vi "LoopselFF_1_or_2cam_eventdriven_CC.VI"() -> ()   [LabVIEW 2015]
uses:
  board.vis/Globals.vi
  <vilib>/Analysis/NI_AALBase.lvlib
panel:
  in  "channel select\n1: CHA\n2: CHB\n3: both CH":u16=3
  out "tRMS":dbl=8.272957184592048 format="%0#.1f"
  out "mean":dbl=3064.5285285285286 format="%#_4f"
  in  "Pixel":u16=100
  in  "is FFT":bool=TRUE
  in  "IR gain":bool
  in  "continuous":bool=TRUE
  out "curr.block":u8=1
  out "Measure ON":bool
  in  "Board select\n1: board 1\n2: board 2\n3: both boards":u8=3
  in  "no.of blocks (nob)\npress enter":u32=1
  in  "NOB":u32(slide)=1 max=10 scale=0.9..1.0
  out "Signalverlaufgraph 2":u16[](graph)=[0, 0, 543, 543, 0, 1, 0, 0, 2, 2, 3, 3, 4, 4, 5, 5, 6, 6, 7, 7, 8, 8, 9, 9, 10, 10, 11, 11, 12, 12, 13, 13, 14, 14, 15, 15, 16, 16, 17, 17, 18, 18, 19, 19, 20, 20, 21, 21, 22, 22, 23, 23, 24, 24, 25, 25, 26, 26, 27, 27, 28, 28, 29, 29, 30, 30, 31, 31, 32, 32, 33, 33, 34, 34, 35, 35, 36, 36, 37, 37, 38, 38, 39, 39, 40, 40, 41, 41, 42, 42, 43, 43, 44, 44, 45, 45, 46, 46, 47, 47, 48, 48, 49, 49, 50, 50, 51, 51, 52, 52, 53, 53, 54, 54, 55, 55, 56, 56, 57, 57, 58, 58, 59, 59, 60, 60, 61, 61, 62, 62, 63, 63, 64, 64, 65, 65, 66, 66, 67, 67, 68, 68, 69, 69, 70, 70, 71, 71, 72, 72, 73, 73, 74, 74, 75, 75, 76, 76, 77, 77, 78, 78, 79, 79, 80, 80, 81, 81, 82, 82, 83, 83, 84, 84, 85, 85, 86, 86, 87, 87, 88, 88, 89, 89, 90, 90, 91, 91, 92, 92, 93, 93, 94, 94, 95, 95, 96, 96, 97, 97, 98, 98, 99, 99, 100, 100, 101, 101, 102, 102, 103, 103, 104, 104, 105, 105, 106, 106, 107, 107, 108, 108, 109, 109, 110, 110, 111, 111, 112, 112, 113, 113, 114, 114, 115, 115, 116, 116, 117, 117, 118, 118, 119, 119, 120, 120, 121, 121, 122, 122, 123, 123, 124, 124, 125, 125, 126, 126, 127, 127, 128, 128, 129, 129, 130, 130, 131, 131, 132, 132, 133, 133, 134, 134, 135, 135, 136, 136, 137, 137, 138, 138, 139, 139, 140, 140, 141, 141, 142, 142, 143, 143, 144, 144, 145, 145, 146, 146, 147, 147, 148, 148, 149, 149, 150, 150, 151, 151, 152, 152, 153, 153, 154, 154, 155, 155, 156, 156, 157, 157, 158, 158, 159, 159, 160, 160, 161, 161, 162, 162, 163, 163, 164, 164, 165, 165, 166, 166, 167, 167, 168, 168, 169, 169, 170, 170, 171, 171, 172, 172, 173, 173, 174, 174, 175, 175, 176, 176, 177, 177, 178, 178, 179, 179, 180, 180, 181, 181, 182, 182, 183, 183, 184, 184, 185, 185, 186, 186, 187, 187, 188, 188, 189, 189, 190, 190, 191, 191, 192, 192, 193, 193, 194, 194, 195, 195, 196, 196, 197, 197, 198, 198, 199, 199, 200, 200, 201, 201, 202, 202, 203, 203, 204, 204, 205, 205, 206, 206, 207, 207, 208, 208, 209, 209, 210, 210, 211, 211, 212, 212, 213, 213, 214, 214, 215, 215, 216, 216, 217, 217, 218, 218, 219, 219, 220, 220, 221, 221, 222, 222, 223, 223, 224, 224, 225, 225, 226, 226, 227, 227, 228, 228, 229, 229, 230, 230, 231, 231, 232, 232, 233, 233, 234, 234, 235, 235, 236, 236, 237, 237, 238, 238, 239, 239, 240, 240, 241, 241, 242, 242, 243, 243, 244, 244, 245, 245, 246, 246, 247, 247, 248, 248, 249, 249, 250, 250, 251, 251, 252, 252, 253, 253, 254, 254, 255, 255, 256, 256, 257, 257, 258, 258, 259, 259, 260, 260, 261, 261, 262, 262, 263, 263, 264, 264, 265, 265, 266, 266, 267, 267, 268, 268, 269, 269, 270, 270, 271, 271, 272, 272, 273, 273, 274, 274, 275, 275, 276, 276, 277, 277, 278, 278, 279, 279, 280, 280, 281, 281, 282, 282, 283, 283, 284, 284, 285, 285, 286, 286, 287, 287, 288, 288, 289, 289, 290, 290, 291, 291, 292, 292, 293, 293, 294, 294, 295, 295, 296, 296, 297, 297, 298, 298, 299, 299, 300, 300, 301, 301, 302, 302, 303, 303, 304, 304, 305, 305, 306, 306, 307, 307, 308, 308, 309, 309, 310, 310, 311, 311, 312, 312, 313, 313, 314, 314, 315, 315, 316, 316, 317, 317, 318, 318, 319, 319, 320, 320, 321, 321, 322, 322, 323, 323, 324, 324, 325, 325, 326, 326, 327, 327, 328, 328, 329, 329, 330, 330, 331, 331, 332, 332, 333, 333, 334, 334, 335, 335, 336, 336, 337, 337, 338, 338, 339, 339, 340, 340, 341, 341, 342, 342, 343, 343, 344, 344, 345, 345, 346, 346, 347, 347, 348, 348, 349, 349, 350, 350, 351, 351, 352, 352, 353, 353, 354, 354, 355, 355, 356, 356, 357, 357, 358, 358, 359, 359, 360, 360, 361, 361, 362, 362, 363, 363, 364, 364, 365, 365, 366, 366, 367, 367, 368, 368, 369, 369, 370, 370, 371, 371, 372, 372, 373, 373, 374, 374, 375, 375, 376, 376, 377, 377, 378, 378, 379, 379, 380, 380, 381, 381, 382, 382, 383, 383, 384, 384, 385, 385, 386, 386, 387, 387, 388, 388, 389, 389, 390, 390, 391, 391, 392, 392, 393, 393, 394, 394, 395, 395, 396, 396, 397, 397, 398, 398, 399, 399, 400, 400, 401, 401, 402, 402, 403, 403, 404, 404, 405, 405, 406, 406, 407, 407, 408, 408, 409, 409, 410, 410, 411, 411, 412, 412, 413, 413, 414, 414, 415, 415, 416, 416, 417, 417, 418, 418, 419, 419, 420, 420, 421, 421, 422, 422, 423, 423, 424, 424, 425, 425, 426, 426, 427, 427, 428, 428, 429, 429, 430, 430, 431, 431, 432, 432, 433, 433, 434, 434, 435, 435, 436, 436, 437, 437, 438, 438, 439, 439, 440, 440, 441, 441, 442, 442, 443, 443, 444, 444, 445, 445, 446, 446, 447, 447, 448, 448, 449, 449, 450, 450, 451, 451, 452, 452, 453, 453, 454, 454, 455, 455, 456, 456, 457, 457, 458, 458, 459, 459, 460, 460, 461, 461, 462, 462, 463, 463, 464, 464, 465, 465, 466, 466, 467, 467, 468, 468, 469, 469, 470, 470, 471, 471, 472, 472, 473, 473, 474, 474, 475, 475, 476, 476, 477, 477, 478, 478, 479, 479, 480, 480, 481, 481, 482, 482, 483, 483, 484, 484, 485, 485, 486, 486, 487, 487, 488, 488, 489, 489, 490, 490, 491, 491, 492, 492, 493, 493, 494, 494, 495, 495, 496, 496, 497, 497, 498, 498, 499, 499, 500, 500, 501, 501, 502, 502, 503, 503, 504, 504, 505, 505, 506, 506, 507, 507, 508, 508, 509, 509, 510, 510, 511, 511, 512, 512, 513, 513, 514, 514, 515, 515, 516, 516, 517, 517, 518, 518, 519, 519, 520, 520, 521, 521, 522, 522, 523, 523, 524, 524, 525, 525, 526, 526, 527, 527, 528, 528, 529, 529, 530, 530, 531, 531, 532, 532, 533, 533, 534, 534, 535, 535, 536, 536, 537, 537, 538, 538, 539, 539, 540, 540, 541, 541]
  out "Signalverlaufgraph":u16[](graph)=[2357, 2347, 2353, 2358, 0, 1, 0, 1, 2411, 2350, 2363, 2362, 2360, 34762, 35034, 35066, 35068, 35077, 35067, 35071, 35078, 35087, 35089, 35073, 35080, 35063, 35067, 35068, 35056, 35053, 35026, 35070, 35060, 35052, 35055, 35054, 35023, 35040, 35048, 35039, 35058, 35037, 35044, 35031, 35053, 35025, 35066, 35061, 35050, 35073, 35076, 35083, 35075, 35070, 35075, 35085, 35086, 35080, 35089, 35095, 35070, 35081, 35104, 35104, 35105, 35092, 35088, 35095, 35088, 35081, 35081, 35088, 35080, 35084, 35070, 35082, 35073, 35056, 35058, 35059, 35053, 35054, 35077, 35067, 35059, 35054, 35062, 35059, 35059, 35062, 35066, 35064, 35074, 35065, 35068, 35067, 35064, 35069, 35062, 35075, 35092, 35065, 35066, 35083, 35080, 35080, 35081, 35105, 35099, 35081, 35093, 35095, 35085, 35101, 35101, 35088, 35100, 35088, 35099, 35088, 35085, 35101, 35074, 35079, 35081, 35069, 35058, 35069, 35068, 35075, 35079, 35072, 35080, 35080, 35067, 35078, 35064, 35073, 35063, 35054, 35076, 35075, 35084, 35082, 35085, 35067, 35059, 35082, 35080, 35097, 35083, 35088, 35093, 35097, 35078, 35088, 35097, 35091, 35100, 35088, 35091, 35092, 35100, 35086, 35085, 35097, 35088, 35086, 35079, 35077, 35080, 35089, 35073, 35075, 35083, 35074, 35085, 35070, 35078, 35081, 35070, 35060, 35084, 35077, 35080, 35075, 35069, 35069, 35061, 35065, 35065, 35085, 35071, 35088, 35086, 35088, 35089, 35090, 35091, 35088, 35079, 35100, 35098, 35102, 35082, 35075, 35088, 35079, 35086, 35082, 35098, 35088, 35092, 35085, 35085, 35084, 35097, 35085, 35074, 35072, 35085, 35088, 35079, 35079, 35080, 35085, 35094, 35077, 35090, 35081, 35083, 35089, 35090, 35083, 35083, 35086, 35087, 35083, 35094, 35098, 35093, 35103, 35102, 35089, 35096, 35096, 35078, 35075, 35103, 35084, 35089, 35095, 35093, 35085, 35094, 35090, 35100, 35080, 35099, 35081, 35086, 35095, 35101, 35083, 35090, 35087, 35078, 35096, 35077, 35091, 35102, 35089, 35093, 35100, 35081, 35086, 35088, 35093, 35079, 35088, 35083, 35083, 35100, 35107, 35081, 35096, 35098, 35091, 35098, 35106, 35087, 35107, 35094, 35101, 35099, 35085, 35088, 35093, 35084, 35089, 35100, 35096, 35094, 35099, 35085, 35094, 35089, 35104, 35088, 35103, 35099, 35088, 35088, 35083, 35092, 35097, 35096, 35095, 35098, 35076, 35100, 35091, 35084, 35090, 35100, 35110, 35101, 35071, 35094, 35088, 35097, 35076, 35103, 35100, 35102, 35101, 35094, 35096, 35103, 35088, 35093, 35099, 35099, 35102, 35099, 35104, 35089, 35085, 35094, 35110, 35093, 35109, 35094, 35101, 35088, 35100, 35090, 35088, 35090, 35086, 35093, 35107, 35091, 35099, 35104, 35088, 35093, 35093, 35098, 35097, 35108, 35087, 35107, 35092, 35094, 35098, 35097, 35092, 35093, 35085, 35095, 35102, 35094, 35093, 35115, 35088, 35106, 35079, 35105, 35099, 35091, 35128, 35094, 35089, 35088, 35109, 35110, 35087, 35110, 35096, 35095, 35097, 35091, 35099, 35085, 35087, 35112, 35089, 35102, 35085, 35089, 35106, 35094, 35097, 35113, 35110, 35087, 35105, 35097, 35094, 35097, 35097, 35098, 35112, 35092, 35101, 35106, 35092, 35094, 35085, 35107, 35088, 35089, 35094, 35081, 35094, 35103, 35107, 35097, 35101, 35086, 35094, 35108, 35086, 35098, 35102, 35102, 35096, 35080, 35085, 35100, 35089, 35088, 35104, 35112, 35100, 35102, 35102, 35097, 35106, 35099, 35081, 35097, 35101, 35109, 35100, 35114, 35098, 35092, 32940, 29697, 29585, 29528, 29434, 29346, 29303, 29248, 29143, 29102, 29112, 29035, 28966, 28956, 28848, 28789, 28725, 28651, 28612, 28562, 28516, 28427, 28371, 28320, 28264, 28200, 28178, 28101, 28056, 27957, 27925, 27901, 27776, 27758, 27701, 27631, 27579, 27545, 27475, 27425, 27382, 27318, 27302, 27222, 27176, 27114, 27069, 27020, 26974, 26944, 26887, 26793, 26807, 26744, 26714, 26624, 26586, 26540, 26466, 26393, 26379, 26282, 26220, 26157, 26029, 25929, 25768, 25543, 2252, 2400, 2386, 2390, 2368, 2373, 2377, 2379, 2379, 2378, 2377, 2380, 2373, 2379, 2386, 2383, 2376, 2381, 2378, 2377, 2376, 2373, 2385, 2377, 2381, 2376, 2379, 2379, 2376, 2376, 2376, 2379, 2384, 2378, 2374, 2380, 2377, 2381, 2380, 2371, 2379, 2376, 2379, 2384, 2380, 2380, 2377, 2368, 2376, 2375, 2378, 2370, 2374, 2375, 2383, 2372, 2379, 2374, 2381, 2369, 2375, 2368, 2373, 2368, 2368, 2372, 2374, 2371, 2368, 2373, 2372, 2370, 2372, 2374, 2375, 2367, 2367, 2370, 2369, 2375, 2372, 2373, 2378, 2372, 2366, 2372, 2370, 2374, 2365, 2373, 2375, 2374, 2370, 2370, 2369, 2369, 2374, 2371, 2373, 2371, 2372, 2371, 2366, 2368, 2370, 2362, 2370, 2372, 2366, 2374, 2369, 2368, 2371, 2368, 2365, 2362, 2375, 2373, 2369, 2366, 2367, 2371, 2362, 2377, 2371, 2367, 2369, 2366, 2371, 2366, 2364, 2366, 2360, 2365, 2374, 2362, 2371, 2373, 2366, 2364, 2367, 2364, 2368, 2360, 2360, 2363, 2367, 2368, 2367, 2371, 2364, 2368, 2366, 2359, 2363, 2365, 2368, 2368, 2358, 2357, 2365, 2364, 2369, 2362, 2364, 2364, 2363, 2358, 2363, 2364, 2359, 2360, 2358, 2370, 2358, 2361, 2363, 2355, 2361, 2369, 2363, 2366, 2365, 2368, 2363, 2360, 2359, 2361, 2359, 2363, 2356, 2365, 2362, 2360, 2368, 2362, 2366, 2370, 2358, 2366, 2364, 2366, 2362, 2363, 2356, 2365, 2363, 2361, 2363, 2367, 2366, 2365, 2357, 2366, 2359, 2361, 2360, 2360, 2363, 2365, 2364, 2360, 2360, 2357, 2355, 2362, 2361, 2361, 2364, 2364, 2361, 2364, 2361, 2363, 2358, 2363, 2357, 2355, 2357, 2365, 2357, 2367, 2365, 2363, 2354, 2360, 2356, 2358, 2362, 2359, 2360, 2362, 2362, 2355, 2360, 2360, 2360, 2361, 2360, 2359, 2357, 2364, 2359, 2361, 2362, 2360, 2359, 2360, 2355, 2355, 2362, 2358, 2358, 2357, 2357, 2360, 2360, 2363, 2353, 2353, 2358, 2358, 2358, 2362, 2360, 2362, 2359, 2356, 2357, 2360, 2355, 2353, 2360, 2362, 2358, 2358, 2350, 2357, 2362, 2354, 2354, 2356, 2360, 2360, 2355, 2361, 2354, 2360, 2356, 2355, 2355, 2362, 2359, 2362, 2363, 2359, 2361, 2358, 2355, 2356, 2354, 2358, 2364, 2356, 2362, 2358, 2354, 2360, 2362, 2361, 2358, 2361, 2362, 2358, 2363, 2359, 2363, 2364, 2356, 2357, 2356, 2354, 2360, 2357, 2355, 2359, 2358, 2356, 2362, 2360, 2357, 2359, 2357, 2357, 2355, 2357, 2357, 2357, 2364, 2360, 2355, 2358, 2355, 2357, 2360, 2353, 2355, 2352, 2362, 2354, 2355, 2360, 2357, 2352, 2359, 2356, 2356, 2358, 2353, 2357, 2356, 2355, 2349, 2361, 2358, 2354, 2358, 2359, 2355, 2360, 2354, 2357, 2357, 2353, 2354, 2359, 2359, 2355, 2349, 2358, 2358, 2355, 2353, 2353, 2357, 2357, 2357, 2354, 2358, 2359, 2354, 2353, 2352, 2358, 2361, 2357, 2350, 2350, 2352, 2360, 2351, 2355, 2354, 2360, 2357, 2355, 2355, 2355, 2350, 2357, 2357, 2358, 2358, 2356, 2353, 2352, 2354, 2353, 2357, 2357, 2353, 2358, 2360, 2361, 2355, 2357, 2361, 2357, 2358, 2356, 2355, 2358, 2354, 2351, 2355, 2352, 2354, 2352, 2354, 2363, 2359, 2358, 2357, 2349, 2358, 2352, 2356, 2355, 2359, 2353, 2353, 2361, 2359, 2359, 2357, 2357, 2349, 2353, 2353, 2350, 2358, 2357, 2356, 2358, 2356, 2356, 2355, 2355, 2355, 2351, 2355, 2357, 2352, 2354, 2348, 2354, 2348, 2354, 2350, 2352, 2353, 2359, 2356, 2351, 2356, 2357, 2352, 2354, 2355, 2359, 2353, 2354, 2352, 2349, 2362, 2353, 2360, 2349, 2357, 2352, 2359, 2348, 2359, 2349, 2358, 2348, 2349, 2351, 2356, 2353, 2358, 2353, 2354, 2360, 2355, 2356, 2358, 2348, 2351, 2354, 2358, 2360, 2360, 2359, 2356, 2356, 2354, 2357, 2350, 2351, 2351]
  out "boards recognised":u8=1
  in  "alloc mem":bool
  out "FREE \nRAM MB":dbl=14941.0
  out "BUILT-IN\nRAM MB":dbl=18096.0
  out "SEC":dbl=5.9999999999999995e-05
  out "MB RAM":dbl
  in  "pos slope":u8=1
  in  "both slopes":u8
  in  "DAT in 10ns":u32
  in  "extTrig  0/1\n0 : internal\n1:  \"I\" input (laser)":u8
  in  "stop all":bool
  in  "start":bool
  in  "NOS":u32(slide)=2 max=3000 scale=0.9..1000.0
  in  "no.of samples (nos)":u32=3
  in  "exposuretime[ms]":dbl=1.0 format="%.3f"
  # "Start with run"
  # "Abort with ESC"
  # "works only for\namount of CH*542\n=amount of pixel"
  # "press Esc to stop measurement"
  # "exit here"
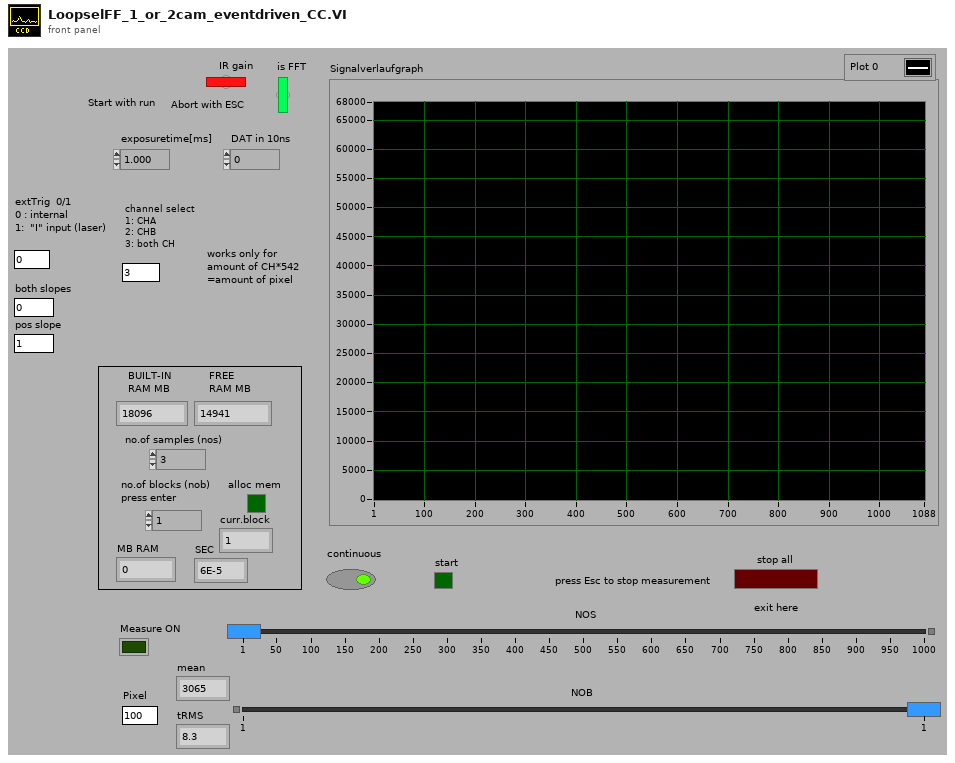
[diagram p1: front panel]
types:
  T1 = enum8{"Enabled", "Disabled", "Disabled and Grayed Out"}
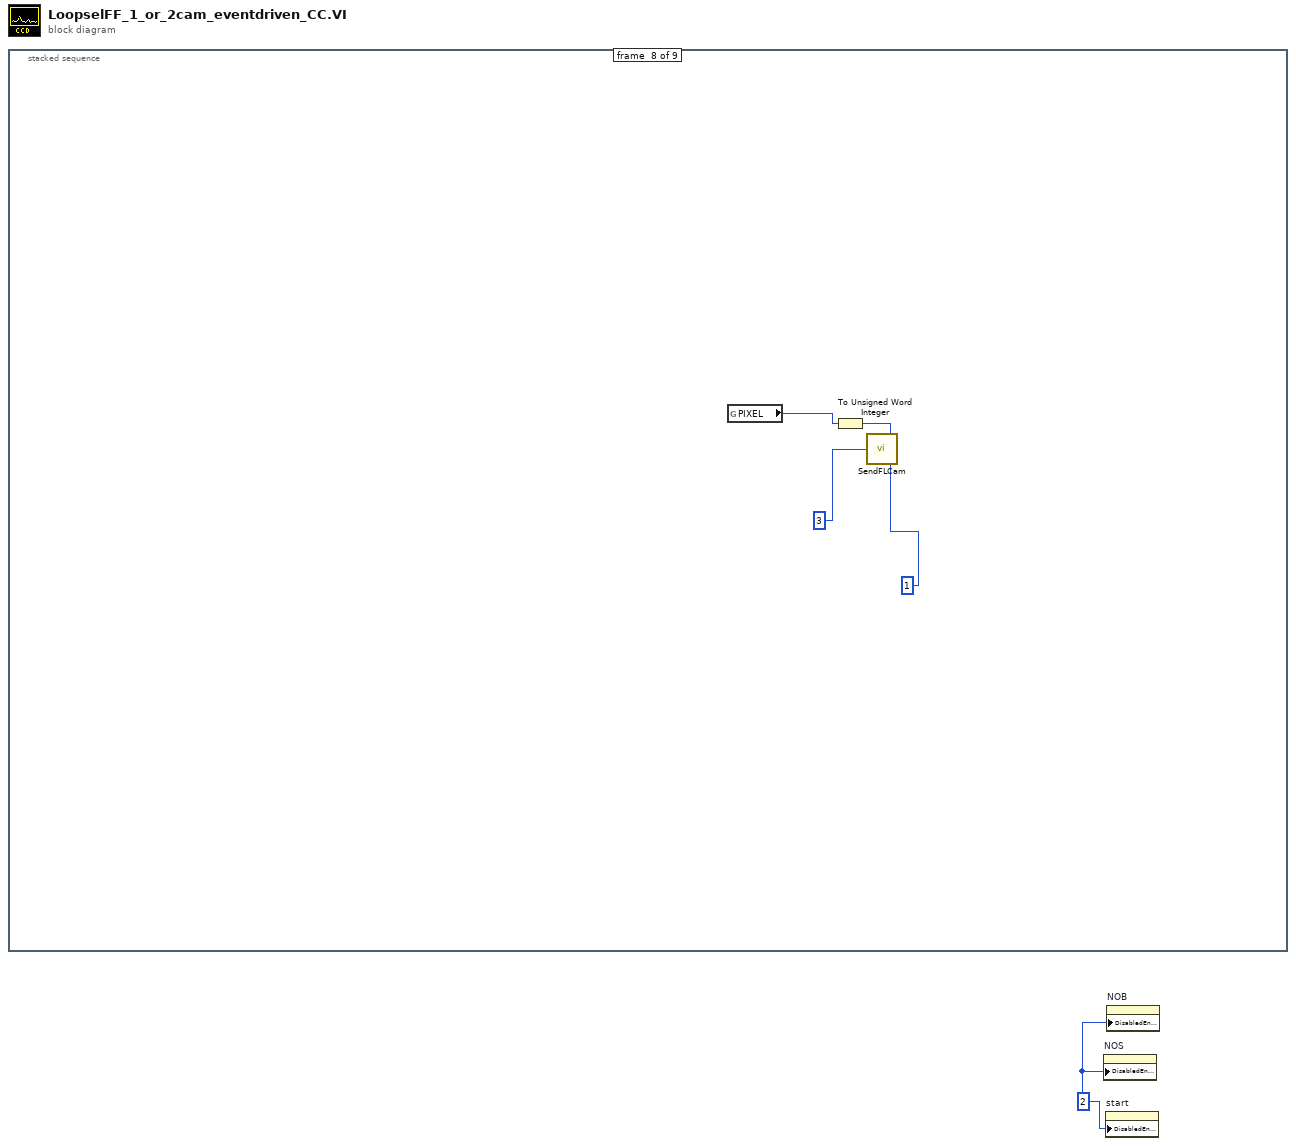
[diagram p0: block diagram]
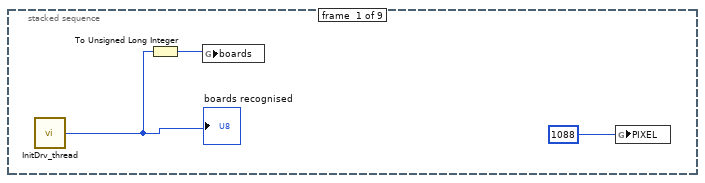
[diagram p2: hidden frame]
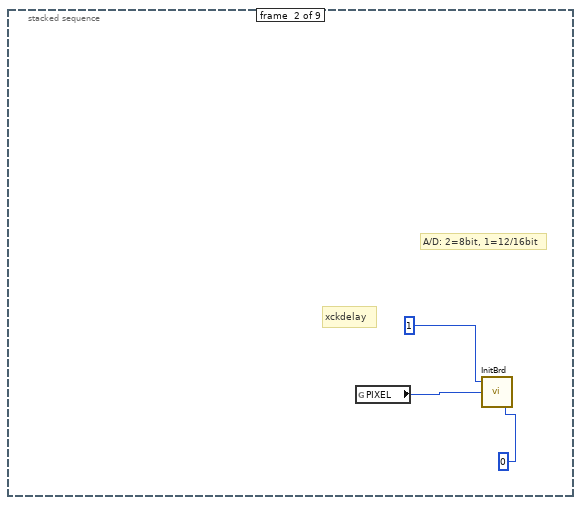
[diagram p3: hidden frame]
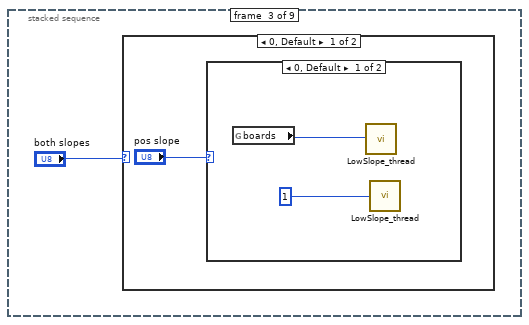
[diagram p4: hidden frame]
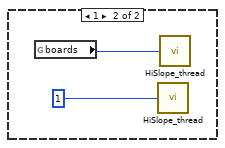
[diagram p5: hidden frame]
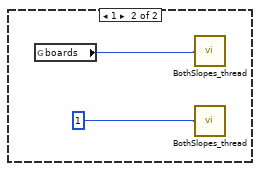
[diagram p6: hidden frame]
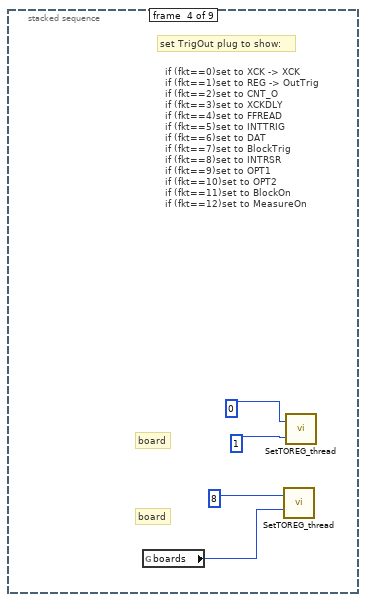
[diagram p7: hidden frame]
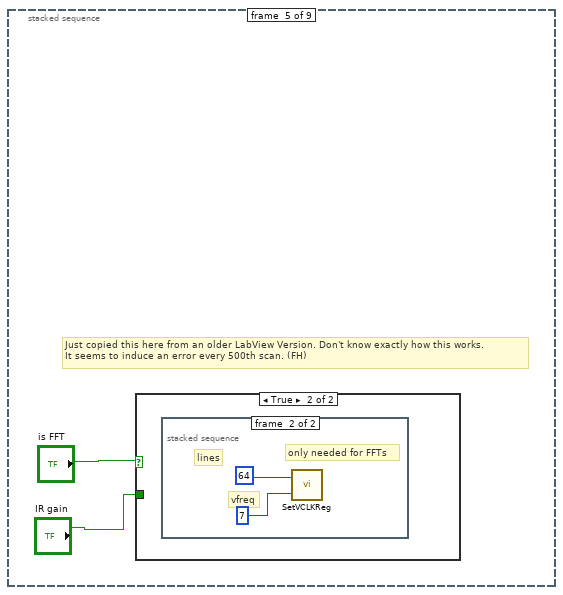
[diagram p8: hidden frame]
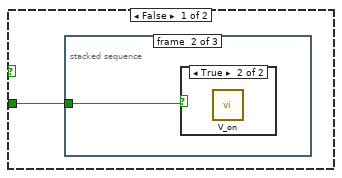
[diagram p9: hidden frame]
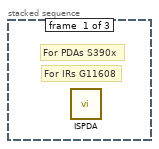
[diagram p10: hidden frame]
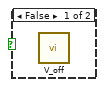
[diagram p11: hidden frame]
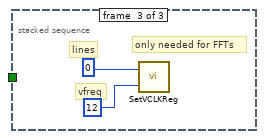
[diagram p12: hidden frame]
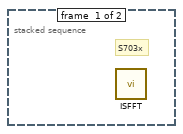
[diagram p13: hidden frame]
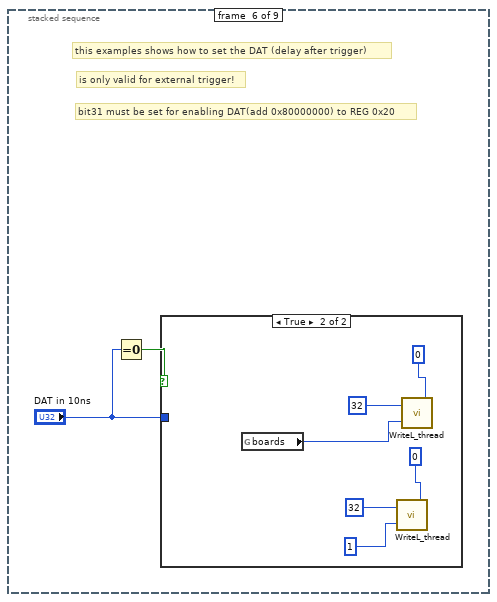
[diagram p14: hidden frame]
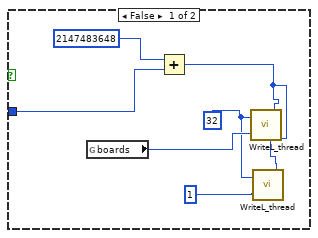
[diagram p15: hidden frame]
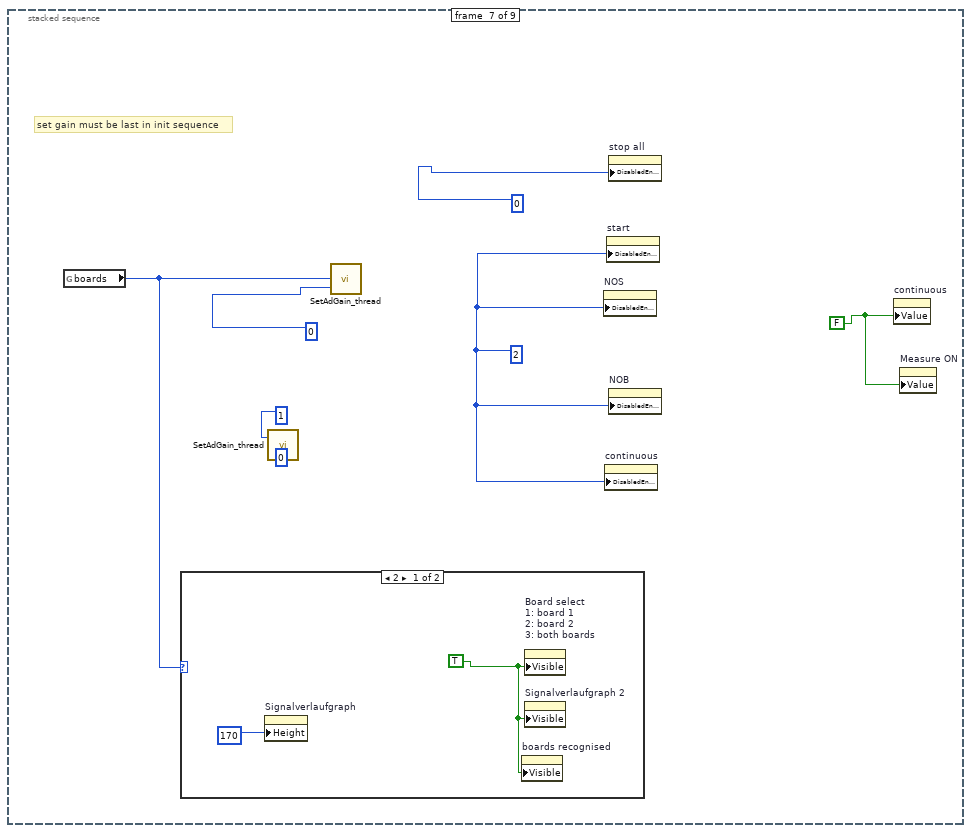
[diagram p16: hidden frame]
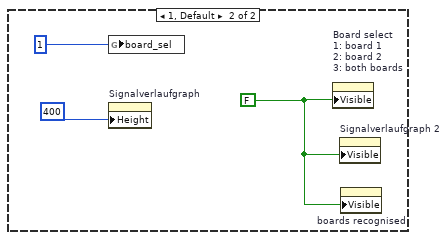
[diagram p17: hidden frame]
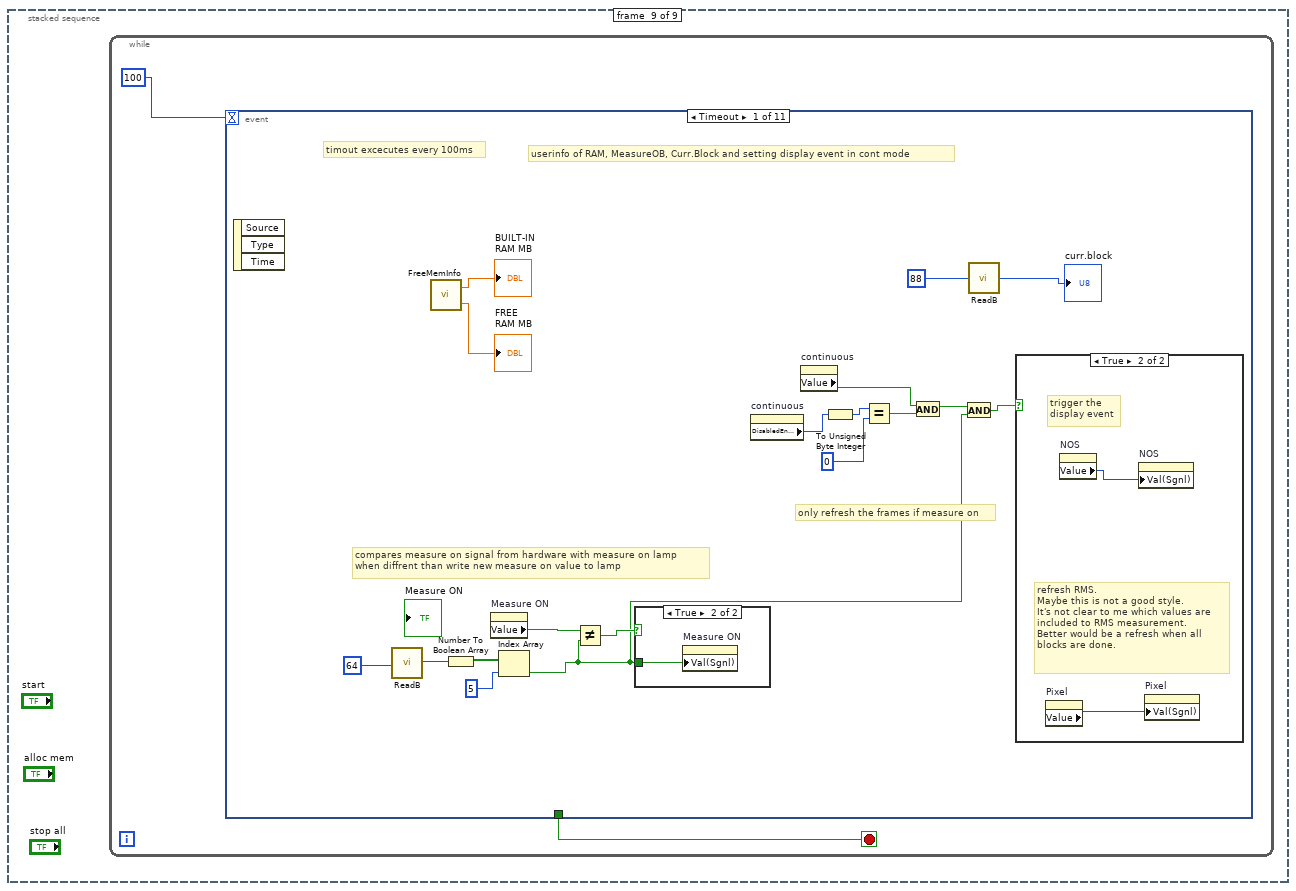
[diagram p18: hidden frame]
diagram:
  w1 = 2
  n1 = stacked-sequence {
    frame #0 {
      n2 = call "InitDrv_thread.vi"() -> ("Boards"=w2:u8)  [unwired: 1 in]
      "boards recognised" <- w2
      n3 = To Unsigned Long Integer(number=w2) -> (unsigned 32bit integer=w3:u32)
      n4 = global write "Globals.vi" "boards"(w3) -> ()
      n5 = global write "Globals.vi" "PIXEL"(u32 1088) -> ()
    }
    frame #1 {
      # "xckdelay"
      # "A/D: 2=8bit, 1=12/16bit"
      n6 = global read "Globals.vi" "PIXEL"() -> (w7:u32)
      n7 = call "InitBrd.vi"("xckdly"=u32 0, "pixel"=w7, "flag816"=u32 1) -> ()  [unwired: 3 in]
    }
    frame #2 {
      n8 = case shown="0, Default" "both slopes" {
        frame 0, Default {
          n9 = case shown="0, Default" "pos slope" {
            frame 0, Default {
              n10 = global read "Globals.vi" "boards"() -> (w10:u32)
              n11 = call "LowSlope_thread.vi"("board"=w10) -> ()  [unwired: 1 in]
              n12 = call "LowSlope_thread.vi"("board"=1) -> ()  [unwired: 1 in]
            }
            frame 1 {
              n13 = global read "Globals.vi" "boards"() -> (w13:u32)
              n14 = call "HiSlope_thread.vi"("board"=1) -> ()  [unwired: 1 in]
              n15 = call "HiSlope_thread.vi"("board"=w13) -> ()  [unwired: 1 in]
            }
          }
        }
        frame 1 {
          n16 = global read "Globals.vi" "boards"() -> (w15:u32)
          n17 = call "BothSlopes_thread.vi"("board"=w15) -> ()  [unwired: 1 in]
          n18 = call "BothSlopes_thread.vi"("board"=1) -> ()  [unwired: 1 in]
        }
      }
    }
    frame #3 {
      # "board"
      # "board"
      # "set TrigOut plug to show:"
      # "if (fkt==0)set to XCK -> XCK\nif (fkt==1)set to REG -> OutTrig\nif (fkt==2)set to CNT_O\nif (fkt==3)set to XCKDLY\nif (fkt==4)set to FFREAD\nif (fkt==5)set to INTTRIG\nif (fkt==6)set to DAT\nif (fkt==7)set to BlockTrig\nif (fkt==8)set to INTRSR\nif (fkt==9)set to OPT1\nif (fkt==10)set to OPT2\nif (fkt==11)set to BlockOn\nif (fkt==12)set to MeasureOn"
      n19 = global read "Globals.vi" "boards"() -> (w19:u32)
      n20 = call "SetTOREG_thread.vi"("board"=w19, "fkt"=u8 8) -> ()  [unwired: 1 in]
      n21 = call "SetTOREG_thread.vi"("board"=u32 1, "fkt"=u8 0) -> ()  [unwired: 1 in]
    }
    frame #4 {
      # "Just copied this here from an older LabView Version. Don't know exactly how this works.\nIt seems to induce an error every 500th scan. (FH)"
      n22 = case shown="True" "is FFT" {
        tunnel: "IR gain" -> [w22 _]
        frame False {
          n23 = stacked-sequence {
            tunnel: w22 -> [_ w23 _]
            frame #0 {
              # "For IRs G11608"
              # "For PDAs S390x"
              n24 = call "ISPDA.vi"() -> ()  [unwired: 1 in]
            }
            frame #1 {
              n25 = case shown="True" w23 {
                frame False {
                  n26 = call "V_off.vi"() -> ()  [unwired: 1 in]
                }
                frame True {
                  n27 = call "V_on.vi"() -> ()  [unwired: 1 in]
                }
              }
            }
            frame #2 {
              # "only needed for FFTs"
              # "vfreq"
              # "lines"
              n28 = call "SetVCLKReg.vi"("vfreq"=u8 12, "lines"=u32 0) -> ()  [unwired: 1 in]
            }
          }
        }
        frame True {
          n29 = stacked-sequence {
            frame #0 {
              # "S703x"
              n30 = call "ISFFT.vi"() -> ()  [unwired: 1 in]
            }
            frame #1 {
              # "only needed for FFTs"
              # "vfreq"
              # "lines"
              n31 = call "SetVCLKReg.vi"("vfreq"=u8 7, "lines"=u32 64) -> ()  [unwired: 1 in]
            }
          }
        }
      }
    }
    frame #5 {
      # "bit31 must be set for enabling DAT(add 0x80000000) to REG 0x20"
      # "is only valid for external trigger!"
      # "this examples shows how to set the DAT (delay after trigger)"
      n32 = Equal To 0?(x="DAT in 10ns") -> (x = 0?=w29:bool)
      n33 = case shown="True" w29 {
        tunnel: "DAT in 10ns" -> [w34 _]
        frame False {
          w31 = u32 32
          n34 = global read "Globals.vi" "boards"() -> (w33:u32)
          n35 = Add(x=u32 2147483648, y=w34) -> (x+y=w32:u32)
          n36 = call "WriteL_thread.vi"("val"=w32, "board"=w33, "offset"=w31) -> ()
          n37 = call "WriteL_thread.vi"("val"=w32, "board"=u32 1, "offset"=w31) -> ()
        }
        frame True {
          n38 = global read "Globals.vi" "boards"() -> (w40:u32)
          n39 = call "WriteL_thread.vi"("val"=u32 0, "board"=u32 1, "offset"=u32 32) -> ()
          n40 = call "WriteL_thread.vi"("val"=u32 0, "board"=w40, "offset"=u32 32) -> ()
        }
      }
    }
    frame #6 {
      w42 = FALSE
      w48 = 2
      # "set gain must be last in init sequence"
      n41 = global read "Globals.vi" "boards"() -> (w46:u32)
      n42 = case shown="2" w46 {
        frame 2 {
          w50 = TRUE
          n43 = property on="Signalverlaufgraph" class="WFGraph (strict)"("Height"=u8 170) -> ()  [unwired: 2 in, 2 out]
          n44 = property on="boards recognised" class="DigNum (strict)"("Visible"=w50) -> ()  [unwired: 2 in, 2 out]
          n45 = property on="Board select\n1: board 1\n2: board 2\n3: both boards" class="DigNum (strict)"("Visible"=w50) -> ()  [unwired: 2 in, 2 out]
          n46 = property on="Signalverlaufgraph 2" class="WFGraph (strict)"("Visible"=w50) -> ()  [unwired: 2 in, 2 out]
        }
        frame 1, Default {
          w51 = FALSE
          n47 = global write "Globals.vi" "board_sel"(u8 1) -> ()
          n48 = property on="Signalverlaufgraph" class="WFGraph (strict)"("Height"=400) -> ()  [unwired: 2 in, 2 out]
          n49 = property on="Board select\n1: board 1\n2: board 2\n3: both boards" class="DigNum (strict)"("Visible"=w51) -> ()  [unwired: 2 in, 2 out]
          n50 = property on="Signalverlaufgraph 2" class="WFGraph (strict)"("Visible"=w51) -> ()  [unwired: 2 in, 2 out]
          n51 = property on="boards recognised" class="DigNum (strict)"("Visible"=w51) -> ()  [unwired: 2 in, 2 out]
        }
      }
      n52 = call "SetAdGain_thread.vi"("gain"=u8 0, "board"=u32 1) -> ()  [unwired: 1 in]
      n53 = call "SetAdGain_thread.vi"("gain"=u8 0, "board"=w46) -> ()  [unwired: 1 in]
      n54 = property on="NOS" class="Slide (strict)"("DisabledEnum"=w48) -> ()  [unwired: 2 in, 2 out]
      n55 = property on="continuous" class="Bool (strict)"("DisabledEnum"=w48) -> ()  [unwired: 2 in, 2 out]
      n56 = property on="start" class="Bool (strict)"("DisabledEnum"=w48) -> ()  [unwired: 2 in, 2 out]
      n57 = property on="stop all" class="Bool (strict)"("DisabledEnum"=0) -> ()  [unwired: 2 in, 2 out]
      n58 = property on="NOB" class="Slide (strict)"("DisabledEnum"=w48) -> ()  [unwired: 2 in, 2 out]
      n59 = property on="continuous" class="Bool (strict)"("Value"=w42) -> ()  [unwired: 2 in, 2 out]
      n60 = property on="Measure ON" class="Bool (strict)"("Value"=w42) -> ()  [unwired: 2 in, 2 out]
    }
    frame #7 {
      n61 = global read "Globals.vi" "PIXEL"() -> (w55:u32)
      n62 = To Unsigned Word Integer(number=w55) -> (unsigned 16bit integer=w54:u16)
      n63 = call "SendFLCam.vi"("madr"=u8 3, "data"=w54, "adadr"=u8 1) -> ()
    }
    frame #8 {
      n64 = while {
        stop <- w59 stop-if-true
        n65 = event shown="[0] Timeout" {
          selector: _ -> [_ _ _ _ _ _ _ _ _ _ _]
          dyn-events: _ -> [_ _ _ _ _ _ _ _ _ _ _]
          timeout: 100 -> [_ _ _ _ _ _ _ _ _ _ _]
          tunnel: [_ _ _ _ _ _ _ _ _ w168 _] -> w59
          event Timeout {
            # "only refresh the frames if measure on"
            # "compares measure on signal from hardware with measure on lamp\nwhen diffrent than write new measure on value to lamp"
            # "timout excecutes every 100ms"
            # "userinfo of RAM, MeasureOB, Curr.Block and setting display event in cont mode"
            n66 = event-data() -> ()  [unwired: 1 in, 3 out]
            n67 = call "ReadB.vi"("Offset"=u32 64) -> ("Data"=w74:u8)
            n68 = call "FreeMemInfo.vi"() -> ("PhysicalSpace"=→"BUILT-IN\nRAM MB":dbl, "PhysicalFreeSpace"=→"FREE \nRAM MB":dbl)  [unwired: 1 in]
            n69 = Number To Boolean Array(number=w74) -> (Boolean array=w73:bool[])
            n70 = property on="Measure ON" class="Bool (strict)"() -> ("Value"=w67:bool)  [unwired: 2 in, 2 out]
            n71 = Index Array(array=w73, index=5) -> (element=w63:bool)
            n72 = Not Equal?(x=w67, y=w63) -> (x != y?=w66:bool)
            n73 = case shown="True" w66 {
              tunnel: w63 -> [_ w78]
              frame False {
              }
              frame True {
                n74 = property on="Measure ON" class="Bool (strict)"("Val(Sgnl)"=w78) -> ()  [unwired: 2 in, 2 out]
              }
            }
            n75 = property on="continuous" class="Bool (strict)"() -> ("DisabledEnum"=w60:T1)  [unwired: 2 in, 2 out]
            n76 = property on="continuous" class="Bool (strict)"() -> ("Value"=w69:bool)  [unwired: 2 in, 2 out]
            n77 = To Unsigned Byte Integer(number=w60) -> (unsigned 8bit integer=w61:u8)
            n78 = Equal?(x=w61, y=u8 0) -> (x = y?=w68:bool)
            n79 = And(x=w69, y=w68) -> (x .and. y?=w65:bool)
            n80 = And(x=w65, y=w63) -> (x .and. y?=w64:bool)
            n81 = call "ReadB.vi"("Offset"=u32 88) -> ("Data"=→"curr.block":u8)
            n82 = case shown="True" w64 {
              frame False {
              }
              frame True {
                # "refresh RMS.\nMaybe this is not a good style.\nIt's not clear to me which values are \nincluded to RMS measurement.\nBetter would be a refresh when all\nblocks are done."
                # "trigger the \ndisplay event"
                n83 = property on="Pixel" class="DigNum (strict)"() -> ("Value"=w79:u16)  [unwired: 2 in, 2 out]
                n84 = property on="NOS" class="Slide (strict)"() -> ("Value"=w80:u32)  [unwired: 2 in, 2 out]
                n85 = property on="NOS" class="Slide (strict)"("Val(Sgnl)"=w80) -> ()  [unwired: 2 in, 2 out]
                n86 = property on="Pixel" class="DigNum (strict)"("Val(Sgnl)"=w79) -> ()  [unwired: 2 in, 2 out]
              }
            }
          }
          event "Measure ON": Value Change {
            # "triggers on value change of measure on. this happens on start of measurement and after measurement\nwhen continuous: not after finishing all blocks, only when exiting measurement"
            n87 = event-data() -> ("NewVal"=w81:bool)  [unwired: 1 in, 5 out]
            n88 = property on="continuous" class="Bool (strict)"() -> ("Value"=w82:bool)  [unwired: 2 in, 2 out]
            n89 = And(x=w82, y=w81) -> (x .and. y?=w83:bool)
            n90 = case shown="False" w81 {
              frame False {
                n91 = property on="stop all" class="Bool (strict)"("DisabledEnum"=0) -> ()  [unwired: 2 in, 2 out]
              }
              frame True {
              }
            }
            n92 = case shown="True" w83 {
              frame False {
              }
              frame True {
                n93 = property on="stop all" class="Bool (strict)"("DisabledEnum"=2) -> ()  [unwired: 2 in, 2 out]
              }
            }
          }
          event "Board select\n1: board 1\n2: board 2\n3: both boards": Value Change {
            # "selecting number of cams"
            n94 = event-data() -> ()  [unwired: 1 in, 6 out]
            n95 = global read "Globals.vi" "boards"() -> (w86:u32)
            n96 = case shown="2" w86 {
              frame 0, Default {
              }
              frame 2 {
                n97 = global write "Globals.vi" "board_sel"("Board select\n1: board 1\n2: board 2\n3: both boards") -> ()
              }
            }
          }
          event "continuous": Value Change {
            # "setting continuos mode"
            n98 = event-data() -> ()  [unwired: 1 in, 6 out]
            n99 = case shown="False" "continuous" {
              tunnel: [u8 0 u8 1] -> w88
              frame False {
              }
              frame True {
              }
            }
            n100 = call "contFFLoop.vi"("Numeric"=w88) -> ()  [unwired: 1 in]
          }
          event "alloc mem": Value Change {
            w96 = 0
            # "update params"
            # "Setup DMA"
            n101 = event-data() -> ()  [unwired: 1 in, 6 out]
            n102 = global read "Globals.vi" "nob"() -> (w94:u32)
            n103 = global read "Globals.vi" "boards"() -> (w97:u32)
            n104 = global read "Globals.vi" "nos"() -> (w93:u32)
            n105 = case shown="2" w97 {
              selector: w97 -> [_ w98]
              tunnel: w93 -> [_ w99]
              tunnel: w94 -> [_ w100]
              frame 1, Default {
              }
              frame 2 {
                # "Setup DMA"
                n106 = call "SetupDMA_thread.vi"("blocks"=w100, "nos"=w99, "Drv"=w98) -> ()  [unwired: 2 in]
              }
            }
            n107 = call "SetupDMA_thread.vi"("blocks"=w94, "nos"=w93, "Drv"=u32 1) -> ()  [unwired: 2 in]
            n108 = property on="continuous" class="Bool (strict)"("DisabledEnum"=w96) -> ()  [unwired: 2 in, 2 out]
            n109 = property on="NOB" class="Slide (strict)"("DisabledEnum"=w96) -> ()  [unwired: 2 in, 2 out]
            n110 = property on="NOS" class="Slide (strict)"("DisabledEnum"=w96) -> ()  [unwired: 2 in, 2 out]
            n111 = property on="exposuretime[ms]" class="DigNum (strict)"() -> ("Value"=w95:dbl)  [unwired: 2 in, 2 out]
            n112 = property on="start" class="Bool (strict)"("DisabledEnum"=w96) -> ()  [unwired: 2 in, 2 out]
            n113 = property on="exposuretime[ms]" class="DigNum (strict)"("Val(Sgnl)"=w95) -> ()  [unwired: 2 in, 2 out]
          }
          event "start": Mouse Down {
            # "start measurement"
            # "only 1st PCI board is used for ext. trig."
            # "ext. block trig\n0: internal: Space\n1: PCI \"I\"\n2: S1\n3: S2"
            # "block trigger 0/1\n0: internal -> next block is started immediately \n1: external -> each block has an own trigger"
            n114 = event-data() -> ()  [unwired: 1 in, 8 out]
            n115 = global read "Globals.vi" "exp time"() -> (w106:dbl)
            n116 = Multiply(x=1000.0, y=w106) -> (x*y=w108:dbl)
            n117 = global read "Globals.vi" "board_sel"() -> (w101:u8)
            n118 = To Unsigned Long Integer(number=w108) -> (unsigned 32bit integer=w103:u32)
            n119 = call "ReadFFLoop_thread.vi"("blocktrigger"=u8 0, "btrig_ch"=u8 0, "ExtTrig"="extTrig  0/1\n0 : internal\n1:  \"I\" input (laser)", "cam_sel"=w101, "exptus"=w103) -> ()  [unwired: 1 in]
          }
          event "NOS", "NOB": Value Change {
            w120 = u32 1
            # "when selecting a value\nbigger than possible\nnos or nob, a dummy \nvalue \"1\" is chosen\n\nTODO:\ninsert error handling\nwith lower values than 1"
            # "display"
            n120 = event-data() -> ()  [unwired: 1 in, 6 out]
            n121 = global read "Globals.vi" "boards"() -> (w123:u32)
            n122 = global read "Globals.vi" "nob"() -> (w112:u32)
            n123 = global read "Globals.vi" "nos"() -> (w119:u32)
            n124 = Greater?(x=w112, y="NOB") -> (0:w115:bool)
            n125 = Greater?(x=w119, y="NOS") -> (0:w118:bool)
            n126 = global read "Globals.vi" "PIXEL"() -> (w109:u32)
            n127 = case shown="False" w115 {
              tunnel: [u32 1 w128] -> w114
              tunnel: "NOB" -> [_ w128]
              frame False {
              }
              frame True {
              }
            }
            n128 = case shown="False" w118 {
              tunnel: [u32 1 w130] -> w117
              tunnel: "NOS" -> [_ w130]
              frame False {
              }
              frame True {
              }
            }
            n129 = To Long Integer(number=w109) -> (32bit integer=w110:i32)
            n130 = Initialize Array(u16 100, w110) -> (w126:u16[])
            n131 = Subtract(x=w117, y=w120) -> (x-y=w122:u32)
            n132 = Subtract(x=w114, y=w120) -> (x-y=w121:u32)
            n133 = case shown="2" w123 {
              selector: w123 -> [_ w135]
              tunnel: w122 -> [_ w136]
              tunnel: w121 -> [_ w133]
              frame 0, Default {
              }
              frame 2 {
                n134 = global read "Globals.vi" "PIXEL"() -> (w131:u32)
                n135 = To Long Integer(number=w131) -> (32bit integer=w132:i32)
                n136 = Initialize Array(u16 100, w132) -> (w138:u16[])
                n137 = call "ReturnFrame.vi"("Data Values In"=w138, "curr_nob"=w133, "curr_nos"=w136, "Drv"=w135) -> ("Data Values Out"=→"Signalverlaufgraph 2":u16[])  [unwired: 1 in]
              }
            }
            n138 = call "ReturnFrame.vi"("Data Values In"=w126, "curr_nob"=w121, "curr_nos"=w122, "Drv"=u32 1) -> ("Data Values Out"=→"Signalverlaufgraph":u16[])  [unwired: 1 in]
          }
          event "channel select\n1: CHA\n2: CHB\n3: both CH": Value Change {
            # "TODO:\nif 3 is choosen for both cam, \nthe complete routine for showing both scans\nseperated in two parts of one scan with the double o9f pixel"
            n139 = event-data() -> ()  [unwired: 1 in, 6 out]
            n140 = case shown="1, 2, Default" "channel select\n1: CHA\n2: CHB\n3: both CH" {
              frame 1, 2, Default {
                n141 = property on="Signalverlaufgraph 2" class="WFGraph (strict)"("Visible"=FALSE) -> ()  [unwired: 2 in, 2 out]
                n142 = property on="Signalverlaufgraph" class="WFGraph (strict)"("Height"=u32 400) -> ()  [unwired: 2 in, 2 out]
              }
              frame 3 {
                n143 = property on="Signalverlaufgraph" class="WFGraph (strict)"("Height"=u32 170) -> ()  [unwired: 2 in, 2 out]
                n144 = property on="Signalverlaufgraph 2" class="WFGraph (strict)"("Visible"=TRUE) -> ()  [unwired: 2 in, 2 out]
              }
            }
            n145 = To Unsigned Byte Integer(number="channel select\n1: CHA\n2: CHB\n3: both CH") -> (unsigned 8bit integer=w140:u8)
            n146 = global write "Globals.vi" "cam_sel"(w140) -> ()
            n147 = call "SendFLCam.vi"("madr"=u8 3, "data"="channel select\n1: CHA\n2: CHB\n3: both CH", "adadr"=u8 2) -> ()
          }
          event "no.of samples (nos)", "no.of blocks (nob)\npress enter", "exposuretime[ms]": Value Change {
            # "calculation of MB RAM an SEC and setting scale max"
            # "MB"
            # "ushort"
            n148 = event-data() -> ()  [unwired: 1 in, 7 out]
            n149 = global read "Globals.vi" "PIXEL"() -> (w167:u32)
            n150 = global read "Globals.vi" "boards"() -> (w166:u32)
            n151 = Multiply(x="no.of samples (nos)", y=w167) -> (x*y=w164:u32)
            n152 = Multiply(x=w164, y=u32 2) -> (x*y=w165:u32)
            n153 = global read "Globals.vi" "nos"() -> (w153:u32)
            n154 = global read "Globals.vi" "nob"() -> (w154:u32)
            n155 = Multiply(x=w165, y=w166) -> (x*y=w152:u32)
            n156 = To Double Precision Float(number=w152) -> (double precision float=w151:dbl)
            n157 = Divide(x=w151, y=1048576.0) -> (x/y=w156:dbl)
            n158 = To Double Precision Float(number="no.of blocks (nob)\npress enter") -> (double precision float=w149:dbl)
            n159 = property on="NOS" class="Slide (strict)"("Scale.Maximum"=w153) -> ()  [unwired: 2 in, 2 out]
            n160 = property on="NOB" class="Slide (strict)"("Scale.Maximum"=w154) -> ()  [unwired: 2 in, 2 out]
            n161 = Multiply(x=w156, y=w149) -> (x*y=→"MB RAM":dbl)
            n162 = global write "Globals.vi" "nos"("no.of samples (nos)") -> ()
            n163 = Multiply(x="no.of samples (nos)", y="no.of blocks (nob)\npress enter") -> (x*y=w147:u32)
            n164 = global write "Globals.vi" "nob"("no.of blocks (nob)\npress enter") -> ()
            n165 = To Double Precision Float(number=w147) -> (double precision float=w148:dbl)
            n166 = global write "Globals.vi" "exp time"("exposuretime[ms]") -> ()
            n167 = Multiply(x="exposuretime[ms]", y=w148) -> (x*y=w162:dbl)
            n168 = Divide(x=w162, y=1000.0) -> (x/y=→"SEC":dbl)
          }
          event "stop all": Value Change {
            # "exit"
            n169 = event-data() -> ()  [unwired: 1 in, 6 out]
            n170 = stacked-sequence {
              tunnel: [_ TRUE] -> w168
              frame #0 {
                n171 = call "FFStop.vi"() -> ()  [unwired: 1 in]
              }
              frame #1 {
                # "do not omit, or next call of driver will go wrong."
                n172 = call "Exit.vi"() -> ()  [unwired: 1 in]
              }
            }
          }
          event "Pixel": Value Change {
            # "one array with all values (except first 10)\nat index Pixel from all blocks"
            n173 = event-data() -> ()  [unwired: 1 in, 6 out]
            n174 = global read "Globals.vi" "nos"() -> (w174:u32)
            n175 = global read "Globals.vi" "nob"() -> (w175:u32)
            n176 = for {
              N: w175 -> [_]
              tunnel: w174 -> [w176]
              tunnel: [w178] -> w171 mode=concatenating
              i -> [w182]
              # "delete first 10 values"
              # "array of all values\nat index Pixel"
              n177 = To Long Integer(number=w176) -> (32bit integer=w177:i32)
              n178 = for {
                N: w177 -> [_]
                tunnel: w182 -> [w187]
                tunnel: [w191] -> w179 mode=indexing
                i -> [w189]
                # "use only value at index \"Pixel\""
                # "init array of size PIXEL\nwith value 100"
                n179 = global read "Globals.vi" "PIXEL"() -> (w183:u32)
                n180 = To Long Integer(number=w183) -> (32bit integer=w184:i32)
                n181 = To Unsigned Long Integer(number=w187) -> (unsigned 32bit integer=w188:u32)
                n182 = To Unsigned Long Integer(number=w189) -> (unsigned 32bit integer=w190:u32)
                n183 = Initialize Array(u16 100, w184) -> (w193:u16[])
                n184 = call "ReturnFrame.vi"("Data Values In"=w193, "curr_nob"=w188, "curr_nos"=w190, "Drv"=u32 1) -> ("Data Values Out"=w192:u16[])  [unwired: 1 in]
                n185 = To Long Integer(number="Pixel") -> (32bit integer=w185:i32)
                n186 = Index Array(array=w192, index=w185) -> (element=w191:u16)
              }
              n187 = Delete From Array(array=w179, length=10, index=0) -> (array with subset deleted=w178:u16[])  [unwired: 1 out]
            }
            n188 = To Double Precision Float(number=w171) -> (double precision float=w170:dbl[])
            n189 = call <vilib>:"Std Deviation and Variance.vi"("X"=w170) -> ("mean"=→"mean":dbl, "standard deviation"=→"tRMS":dbl)  [unwired: 1 in, 1 out]
          }
        }
      }
    }
  }
  n190 = property on="NOS" class="Slide (strict)"("DisabledEnum"=w1) -> ()  [unwired: 2 in, 2 out]
  n191 = property on="start" class="Bool (strict)"("DisabledEnum"=w1) -> ()  [unwired: 2 in, 2 out]
  n192 = property on="NOB" class="Slide (strict)"("DisabledEnum"=w1) -> ()  [unwired: 2 in, 2 out]
